vi "Proportional action.vi"(1 "error":dbl format="%.2f", 2 "Kc":dbl format="%.4f") -> (0 "proportional action":dbl format="%.2f")   [LabVIEW 2012]
doc: "This function calculates the proportional action of the PID controller."
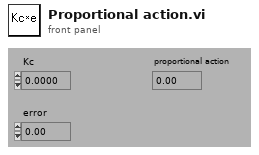
[diagram p1: front panel]
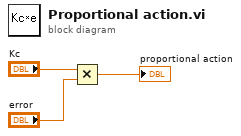
[diagram p0: block diagram]
diagram:
  n1 = Multiply(x="Kc", y="error") -> (x*y=→"proportional action":dbl)
